vi "VI Shut Down Backup.vi"(8 "Fehler (Eingang, kein Fehler)":errorcluster, 11 "VI Referenz":refnum<vi>) -> (0 "Fehler (Ausgang)":errorcluster, 3 "Referenz (Ausgang)":refnum<vi>)   [LabVIEW 2015, in "Backup.lvlib"]
uses:
  Backup.lvlib
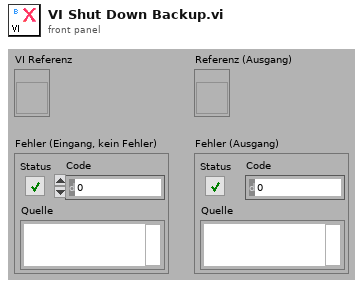
[diagram p1: front panel]
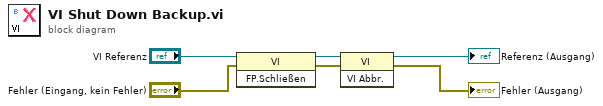
[diagram p0: block diagram]
diagram:
  n1 = invoke class="VI" method="FP.Schließen"(reference="VI Referenz", error in="Fehler (Eingang, kein Fehler)") -> (reference out=w5:refnum<vi>, error out=w4:errorcluster)  [unwired: 1 in, 1 out]
  n2 = invoke class="VI" method="VI Abbr."(reference=w5, error in=w4) -> (reference out=→"Referenz (Ausgang)":refnum<vi>, error out=→"Fehler (Ausgang)":errorcluster)  [unwired: 1 in, 1 out]
